vi "Correção plasticidade.vi"(1 "Sesc":dbl=1401.29 caption="Tensão de escoamento [MPa]", 2 "R":dbl=0.06009682, 3 "Infos para processamento":T1={"Diâmetro do furo [mm]"=1.4, "Diâmetro da linha média [mm]"=5.0, "IncF"=0.2, "Módulo de elasticidade [GPa]"=207.0, "Módulo de Poisson"=0.3, "Tipo de roseta utilizada"=enum."Tipo A", "Método de análise"=enum."Simplificado 2008", "Pfinal"=0.3, "Parar auto."=TRUE}, 4 "Resultados":dbl[][](array[numeric])=[[0.05, 62.82873799168597, -23.97645851949176, 47.11711194337758, -8.264832471183373, -33.421484011809916, 25.17847899224649, 77.64490653645292], [0.1, -423.77374582652806, -1019.9621765762014, -424.72967304368325, -1019.0062493590461, 23.853698888478277, -2.294876929221599, 887.509908186288], [0.15, -865.3188670037671, -1892.5660906600895, -876.0148889472873, -1881.870068716569, 104.27393710909726, -5.856698259156142, 1641.0088372124508], [0.2, -1216.6699924342183, -2450.530487550347, -1244.2012293534453, -2422.9992506311205, 182.24087524486438, -8.590746784929076, 2122.2390607930865], [0.25, -1421.9067969749156, -2737.234228360495, -1473.22615922158, -2685.9148661138306, 254.69214354362597, -11.392307916143091, 2371.113284086942], [0.3, -1469.1923094620595, -2841.0601542026743, -1547.436435981421, -2762.8160276833128, 318.14848400856886, -13.816875160630433, 2460.911439427864], [0.35, -1394.5409609401013, -2749.5133325739307, -1495.314105597265, -2648.7401879167664, 355.5131504305044, -15.82582043142515, 2381.230583714285], [0.4, -1242.2181616608052, -2532.103871451614, -1354.3822397562058, -2419.9397933562136, 363.45296954644135, -17.150584523095258, 2192.995795858116], [0.45, -1041.663952485838, -2233.445853587227, -1146.197757710314, -2128.9120483627507, 337.12635714977756, -17.227255762813286, 1935.6766608355895], [0.5, -811.5545677472688, -2006.178288740522, -919.8112468072139, -1897.921609680577, 342.93802384669453, -17.519561289642166, 1747.9270547429992], [0.55, -593.1664130311339, -1799.5102712440473, -709.272967262429, -1683.4037170127522, 355.78602650992735, -18.073480091862574, 1588.2929695287744], [0.6, -403.9502911130825, -1585.996367506975, -518.4440397278311, -1471.5026188922266, 349.6113096709473, -18.13303600729013, 1427.5491659053043], [0.65, -242.88184795123468, -1383.849147285057, -349.9597530496471, -1276.7712421866447, 332.72617937005555, -17.839208384266776, 1279.8117894157135], [0.7, -121.66118106203376, -1171.1145707642306, -211.96570298185378, -1080.8100488444106, 294.3050797302422, -17.058099431038187, 1115.2719843139448], [0.75, -36.989119056463004, -938.2249880519936, -104.370181699629, -870.8439254088275, 237.03591065940566, -15.868606676508955, 920.2881110548658], [0.8, 36.36379231254571, -712.5972584899445, -5.705561409533024, -670.5279047678656, 172.44847592158175, -13.709704864677303, 731.4573924084386], [0.85, 117.31255341218518, -512.2579793785662, 96.14931147116135, -491.0947374375424, 113.47189385453844, -10.564653415712241, 579.8834056875265], [0.9, 212.58621303943585, -342.040065632566, 204.73699100519607, -334.1908435983262, 65.51163652953481, -6.832276774041858, 484.6620541500704], [0.95, 319.0150500364392, -194.02706349938327, 318.0635680813417, -193.07558154428577, 22.073626691677568, -2.468202190993293, 448.68101908886746], [1.0, 439.585109667837, -66.51068858650771, 439.0489582747345, -65.97453719340515, -16.463793881153105, 1.865205540143952, 476.33585701091096]]) -> (0 "Comparação":cluster{"Resultados":dbl[], dbl[]}[](graph))   [LabVIEW 2018]
uses:
  Controles/Infos para processamento.ctl
panel:
  out "i":i32
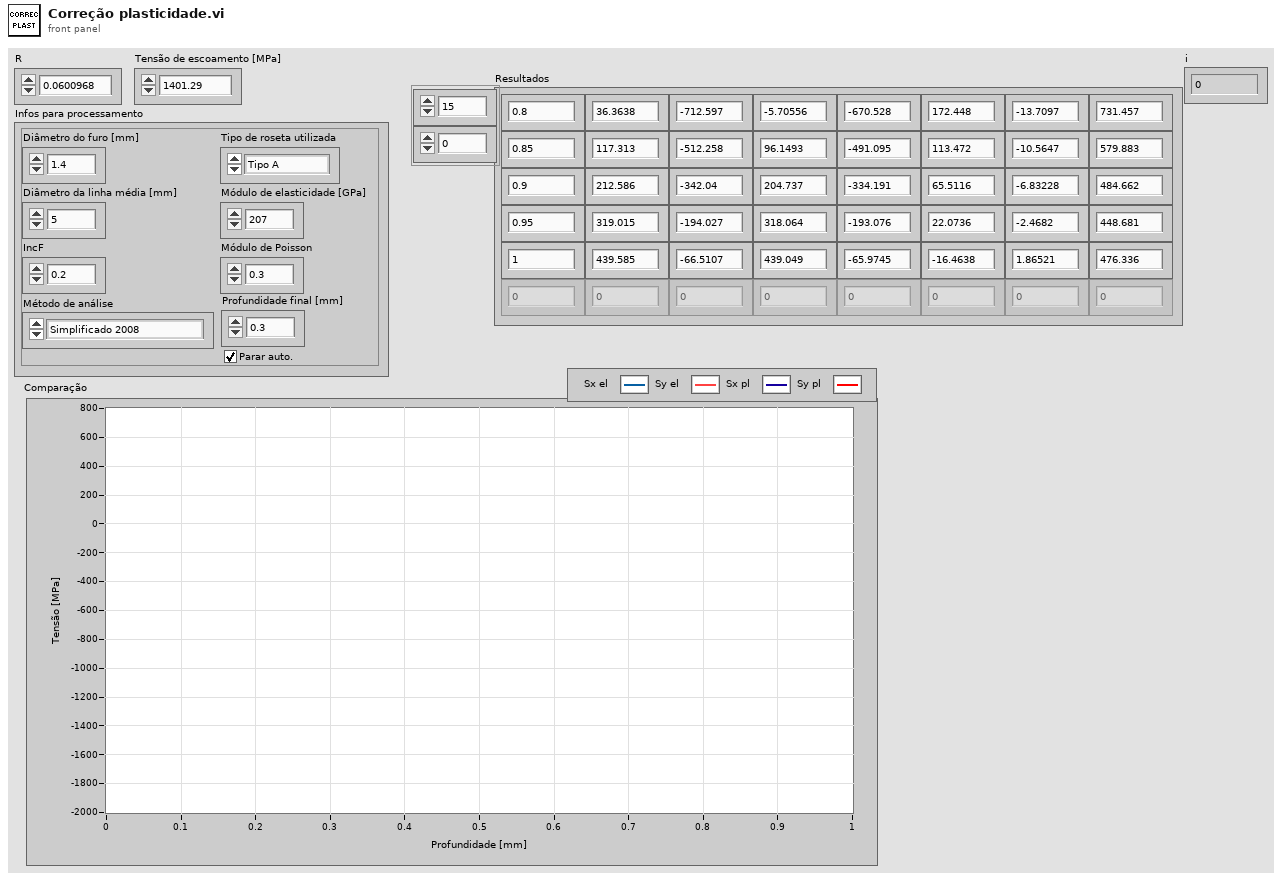
[diagram p1: front panel]
types:
  T1 = typedef "Infos para processamento.ctl" = cluster{"Diâmetro do furo [mm]":dbl, "Diâmetro da linha média [mm]":dbl, "IncF":dbl, "Módulo de elasticidade [GPa]":dbl, "Módulo de Poisson":dbl, "Tipo de roseta utilizada":enum16{"Tipo A", "Tipo B", "Tipo C"}, "Método de análise":enum16{"Não uniforme 2013", "Simplificado 2013", "Simplificado 2008"}, "Pfinal":dbl, "Parar auto.":bool}
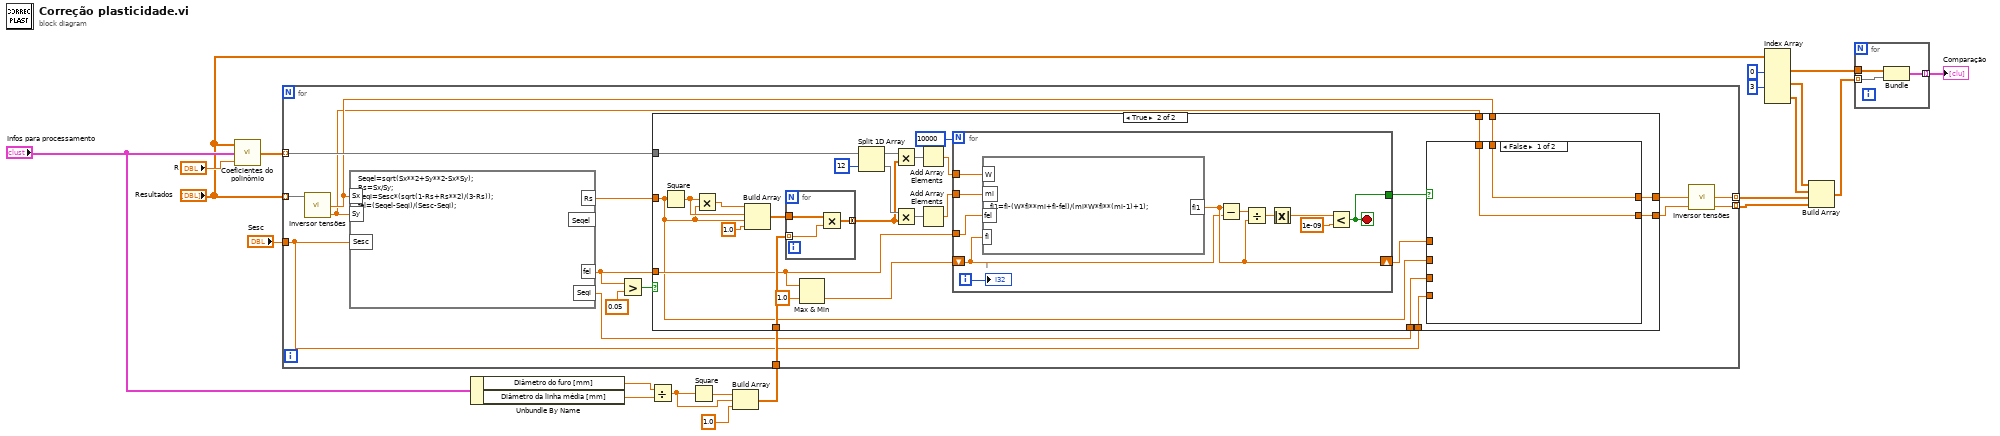
[diagram p0: block diagram]
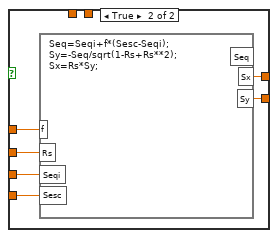
[diagram p3: hidden frame]
diagram:
  n1 = call "Coeficientes do polinômio.vi"("R"="R", "Infos para processamento"="Infos para processamento", "Resultados"="Resultados") -> ("Coeficientes"=w19:dbl[][])
  n2 = Unbundle By Name("Infos para processamento") -> ("Diâmetro do furo [mm]"=w15:dbl, "Diâmetro da linha média [mm]"=w16:dbl)
  n3 = Divide(x=w15, y=w16) -> (x/y=w13:dbl)
  n4 = Square(x=w13) -> (x^2=w14:dbl)
  n5 = Build Array(w14, w13, 1.0 ("element")) -> (w11:dbl[])
  n6 = for {
    tunnel: w19 -> [w34] mode=indexing
    tunnel: "Resultados" -> [w31] mode=indexing
    tunnel: "Sesc" -> [w33]
    tunnel: w11 -> [w35]
    tunnel: [w26] -> w10 mode=indexing
    tunnel: [w25] -> w9 mode=indexing
    n7 = call "Inversor tensões.vi"("Dados"=w31) -> ("Out 2"=w29:dbl, "Out 1"=w30:dbl)  [unwired: 3 in]
    n8 = formula code="Seqel=sqrt(Sx**2+Sy**2-Sx*Sy);\nRs=Sx/Sy;\nSeqi=Sesc*(sqrt(1-Rs+Rs**2)/(3-Rs));\nfel=(Seqel-Seqi)/(Sesc-Seqi);"("Sx"=w30, "Sy"=w29, "Sesc"=w33) -> ("Rs"=w24:dbl, "Seqi"=w32:dbl, "fel"=w23:dbl)  [unwired: 1 out]
    n9 = Greater?(x=w23, y=0.05) -> (0:w21:bool)
    n10 = case shown="True" w21 {
      tunnel: w24 -> [_ w44]
      tunnel: w35 -> [_ w60]
      tunnel: w34 -> [_ w59]
      tunnel: w23 -> [_ w48]
      tunnel: w33 -> [_ w46]
      tunnel: w32 -> [_ w45]
      tunnel: [w37 w43] -> w28
      tunnel: [w36 w42] -> w27
      tunnel: w30 -> [w37 w39]
      tunnel: w29 -> [w36 w38]
      frame False {
      }
      frame True {
        n11 = Square(x=w44) -> (x^2=w63:dbl)
        n12 = Multiply(x=w63, y=w44) -> (x*y=w64:dbl)
        n13 = Build Array(w64, w63, w44, 1.0 ("element")) -> (w61:dbl[])
        n14 = for {
          tunnel: w61 -> [w86]
          tunnel: w60 -> [w85] mode=indexing
          tunnel: [w84] -> w55 mode=concatenating
          n15 = Multiply(x=w86, y=w85) -> (x*y=w84:dbl[])
        }
        n16 = Max & Min(x=w48, y=1.0) -> (min(x,y)=w51:dbl)  [unwired: 1 out]
        n17 = Split 1D Array(array=w59, index=12) -> (first subarray=w57:dbl[], second subarray=w56:dbl[])
        n18 = Multiply(x=w57, y=w55) -> (x*y=w54:dbl[])
        n19 = Multiply(x=w56, y=w55) -> (x*y=w53:dbl[])
        n20 = Add Array Elements(numeric array=w54) -> (sum=w49:dbl)
        n21 = Add Array Elements(numeric array=w53) -> (sum=w50:dbl)
        n22 = for {
          N: 10000 -> [_]
          shift-right: [w79] -> w47
          shift-left: w51 -> [w76]
          tunnel: w50 -> [w83]
          tunnel: w49 -> [w82]
          tunnel: w48 -> [w81]
          tunnel: [w74] -> w40
          i -> [w73]
          stop <- w74 stop-if-true
          n23 = formula code="fi1=fi-(W*fi**mi+fi-fel)/(mi*W*fi**(mi-1)+1);"("W"=w82, "mi"=w83, "fi"=w76, "fel"=w81) -> ("fi1"=w79:dbl)
          n24 = Subtract(x=w79, y=w76) -> (x-y=w80:dbl)
          n25 = Divide(x=w80, y=w79) -> (x/y=w78:dbl)
          n26 = Absolute Value(x=w78) -> (abs(x)=w75:dbl)
          n27 = Less?(x=w75, y=1e-09) -> (x < y?=w74:bool)
          "i" <- w73
        }
        n28 = case shown="False" w40 {
          tunnel: w47 -> [_ w72]
          tunnel: w46 -> [_ w71]
          tunnel: w45 -> [_ w70]
          tunnel: w44 -> [_ w69]
          tunnel: [w66 w68] -> w43
          tunnel: [w65 w67] -> w42
          tunnel: w39 -> [w66 _]
          tunnel: w38 -> [w65 _]
          frame False {
          }
          frame True {
            n29 = formula code="Seq=Seqi+f*(Sesc-Seqi);\nSy=-Seq/sqrt(1-Rs+Rs**2);\nSx=Rs*Sy;"("f"=w72, "Sesc"=w71, "Seqi"=w70, "Rs"=w69) -> ("Sx"=w68:dbl, "Sy"=w67:dbl)  [unwired: 1 out]
          }
        }
      }
    }
    n30 = call "Inversor tensões.vi"("In 2"=w27, "In 1"=w28) -> ("Out 2"=w25:dbl, "Out 1"=w26:dbl)  [unwired: 2 in]
  }
  n31 = Index Array(array="Resultados", index (col) #1=0 ("disabled index (col)"), index (col) #2=3 ("disabled index (col)")) -> (element #1=w3:dbl[], element #2=w5:dbl[], element #3=w6:dbl[])  [unwired: 4 in]
  n32 = Build Array(w5, w6, w10, w9) -> (w4:dbl[][])
  n33 = for {
    tunnel: w4 -> [w89] mode=indexing
    tunnel: w3 -> [w88]
    tunnel: [w87] -> w2 mode=indexing
    n34 = Bundle("Resultados"=w88, w89) -> (w87:cluster{"Resultados":dbl[], dbl[]})  [unwired: 1 in]
  }
  "Comparação" <- w2
